vi "Move To Origin.vi"(6 "Variant in":variant, 7 "Shift Pressed?":bool, 8 "error in (no error)":errorcluster, 10 "QD Combo Box Ref":refnum<vi>, 11 "QD Launch VI Ref":refnum<vi>) -> (0 "error out":errorcluster, 4 "Variant out":variant)   [LabVIEW 2019]
doc: "Moves everything on the block diagram so that the top left thing on the diagram is 100 right and down from the origin.\n\nDefault Shortcut - [@]"
uses:
  <vilib>/Utility/miscctls.llb/LVDeltaXY32Cluster.ctl
panel:
  in  "Undo Name":string="Move to Origin"
  # "Do not change the connector pane of this VI.\n\nSee the block diagram for directions on how to use this template."
  # "Specify the name of the Undo transaction"
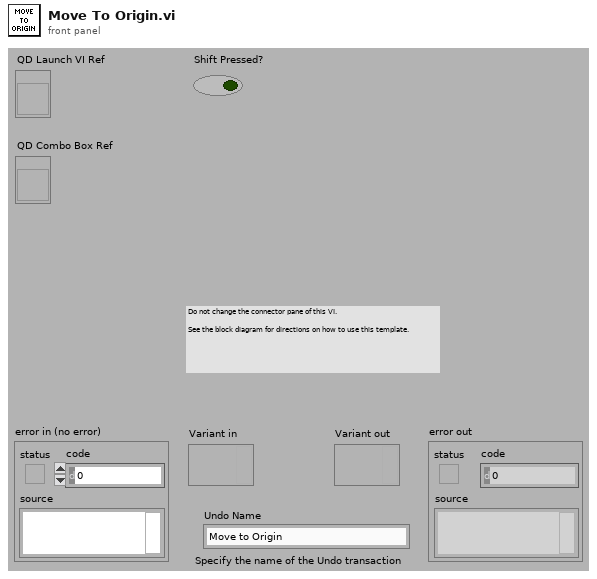
[diagram p1: front panel]
types:
  T1 = typedef "LVDeltaXY32Cluster.ctl" = cluster{"X":i32, "Y":i32}
  T2 = typedef "LVPositionTypeDef.ctl" = cluster{"Left":i32, "Top":i32}
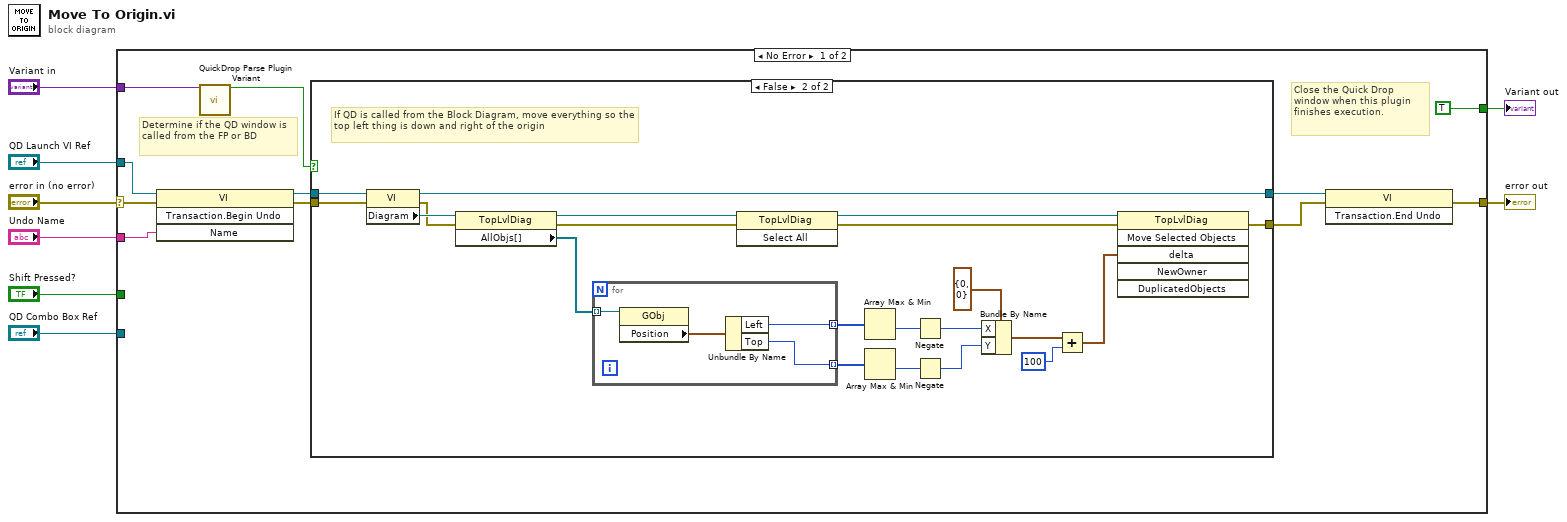
[diagram p0: block diagram]
diagram:
  n1 = case shown="No Error" "error in (no error)" {
    selector: "error in (no error)" -> [w18 w47]
    tunnel: [w12 w47] -> w7
    tunnel: "QD Launch VI Ref" -> [w17 _]
    tunnel: "Shift Pressed?" -> [_ _]
    tunnel: "QD Combo Box Ref" -> [_ _]
    tunnel: "Variant in" -> [w19 _]
    tunnel: "Undo Name" -> [w16 _]
    tunnel: [TRUE _] -> w1
    frame No Error {
      # "Close the Quick Drop window when this plugin finishes execution."
      # "Determine if the QD window is called from the FP or BD"
      n2 = invoke class="VI" method="Transaction.Begin Undo"(reference=w17, error in=w18, "Name"=w16) -> (reference out=w11:refnum<vi>, error out=w13:errorcluster)  [unwired: 1 in, 2 out]
      n3 = call <vilib>:"QuickDrop Parse Plugin Variant.vi"("QDKS Variant in"=w19) -> ("QD Launch VI Panel?"=w14:bool)  [unwired: 12 in, 2 out]
      n4 = case shown="False" w14 {
        tunnel: w13 -> [w21 w42]
        tunnel: w11 -> [w20 w41]
        tunnel: [w21 w27] -> w10
        tunnel: [w20 w40] -> w9
        frame True {
          # "Do nothing on front panel"
        }
        frame False {
          # "If QD is called from the Block Diagram, move everything so the top left thing is down and right of the origin"
          n5 = property class="VI"(reference=w41, error in=w42) -> (reference out=w40:refnum<vi>, error out=w30:errorcluster, "Diagram"=w39:refnum<vi>)
          n6 = property class="TopLvlDiag"(reference=w39, error in=w30) -> (reference out=w26:refnum<vi>, error out=w29:errorcluster, "AllObjs[]"=w38:refnum<vi>[])
          n7 = for {
            tunnel: w38 -> [w46] mode=indexing
            tunnel: [w44] -> w37 mode=indexing
            tunnel: [w43] -> w36 mode=indexing
            n8 = property class="GObj"(reference=w46) -> ("Position"=w45:T2)  [unwired: 1 in, 2 out]
            n9 = Unbundle By Name(w45) -> ("Left"=w44:i32, "Top"=w43:i32)
          }
          n10 = invoke class="TopLvlDiag" method="Select All"(reference=w26, error in=w29) -> (reference out=w35:refnum<vi>, error out=w28:errorcluster)  [unwired: 1 in, 1 out]
          n11 = Array Max & Min(array=w37) -> (min value=w23:i32)  [unwired: 3 out]
          n12 = Array Max & Min(array=w36) -> (min value=w22:i32)  [unwired: 3 out]
          n13 = Negate(x=w23) -> (-x=w32:i32)
          n14 = Negate(x=w22) -> (-x=w31:i32)
          n15 = Bundle By Name(cluster=T1 {"X"=0, "Y"=0} ("X/Y Delta"), "X"=w32, "Y"=w31) -> (w33:T1)
          n16 = Add(x=w33, y=100) -> (x+y=w25:T1)
          n17 = invoke class="TopLvlDiag" method="Move Selected Objects"(reference=w35, error in=w28, "delta"=w25) -> (error out=w27:errorcluster)  [unwired: 3 in, 5 out]
        }
      }
      n18 = invoke class="VI" method="Transaction.End Undo"(reference=w9, error in=w10) -> (error out=w12:errorcluster)  [unwired: 1 in, 2 out]
    }
    frame Error {
    }
  }
  "error out" <- w7
  "Variant out" <- w1
